vi "SaveMainFile.vi"(11 ".NET Refnum in":refnum<k24>) -> (3 "source":string)   [LabVIEW 2017]
uses:
  System.Windows.Forms
panel:
  in  ".NET Refnum in 2":refnum<k24>
  out "source 2":string
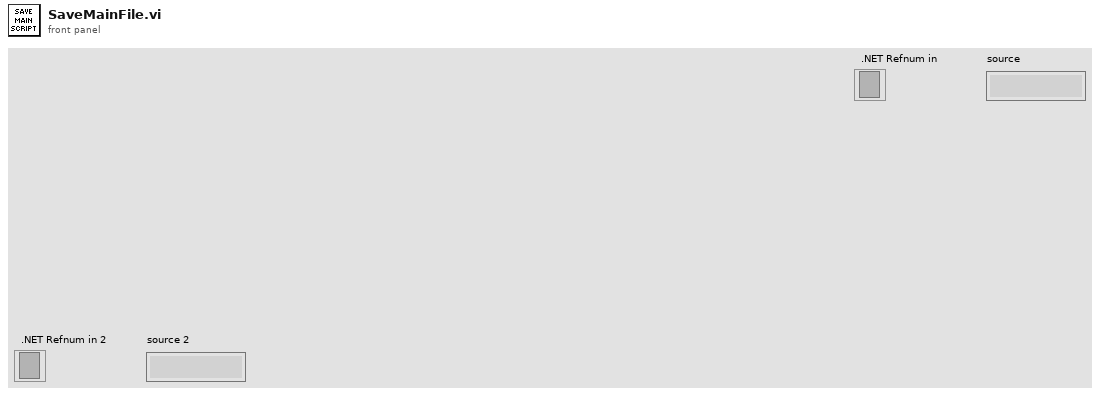
[diagram p1: front panel]
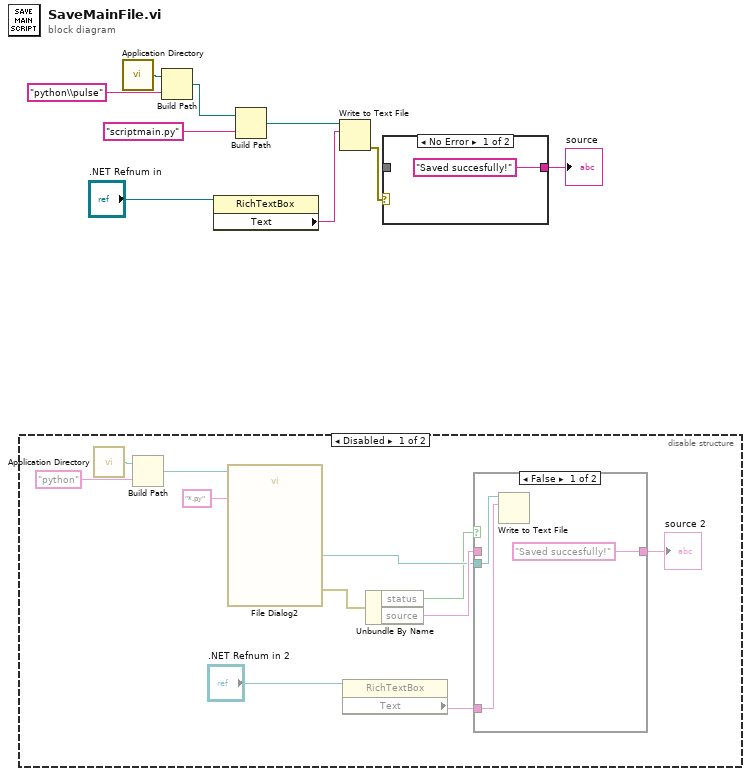
[diagram p0: block diagram]
diagram:
  n1 = disable-structure shown="Disabled" {
    frame Disabled {
      n2 = call <vilib>:"Application Directory.vi"() -> ("Application Directory"=w10:path)
      n3 = Build Path(base path=w10, name or relative path="python") -> (appended path=w12:path)
      n4 = call "File Dialog2"("start path"=w12, "pattern (all files)"="*.py") -> ("selected path"=w16:path, "error out"=w14:errorcluster)  [unwired: 10 in, 2 out]
      n5 = property class="RichTextBox"(reference=".NET Refnum in 2") -> ("Text"=w18:string)  [unwired: 1 in, 2 out]
      n6 = Unbundle By Name(w14) -> ("status"=w15:bool, "source"=w19:string)
      n7 = case shown="False" w15 {
        tunnel: w16 -> [w23 _]
        tunnel: w18 -> [w22 _]
        tunnel: w19 -> [_ w24]
        tunnel: ["Saved succesfully!" ("source") w24] -> w20
        frame False {
          n8 = Write to Text File(file (use dialog)=w23, text=w22) -> ()  [unwired: 2 in, 3 out]
        }
        frame True {
        }
      }
      "source 2" <- w20
    }
    frame Enabled {
    }
  }
  n9 = call <vilib>:"Application Directory.vi"() -> ("Application Directory"=w6:path)
  n10 = Build Path(base path=w6, name or relative path="python\\pulse") -> (appended path=w3:path)
  n11 = property class="RichTextBox"(reference=".NET Refnum in") -> ("Text"=w4:string)  [unwired: 1 in, 2 out]
  n12 = Build Path(base path=w3, name or relative path="scriptmain.py" ("pattern (all files)")) -> (appended path=w1:path)
  n13 = Write to Text File(file (use dialog)=w1, text=w4) -> (error out=w5:errorcluster)  [unwired: 2 in, 2 out]
  n14 = case shown="No Error" w5 {
    tunnel: _ -> [_ w26]
    tunnel: ["Saved succesfully!" ("source") w26] -> w9
    frame No Error {
    }
    frame Error {
    }
  }
  "source" <- w9
